vi "Wait.vi"(4 "error in (no error)":errorcluster, 6 "Delay (0ms)":i32 min=0 max=60000, 7 "VISA resource name":refnum<visa-resource-name>) -> (0 "error out":errorcluster, 3 "VISA resource name out":refnum<visa-resource-name>)   [LabVIEW 2015, in "Newport ESP301.lvlib"]
doc: "This command causes the controller to pause for a specified amount of time. This means that the controller will wait <B>Delay (0ms)</B> milliseconds before executing the next command.\nNote:\nEven though this command can be executed in immediate mode, its real value is as a flow control instruction inside programs.\nWait commands are primarily intended for use in internal program execution or in combination with the RQ command. If used in command mode, it is important to note that input command processing is suspended until the wait condition has been satisfied."
uses:
  Newport ESP301.lvlib
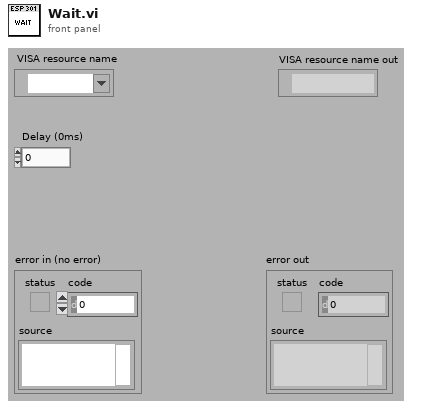
[diagram p1: front panel]
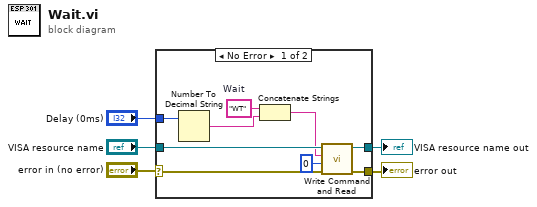
[diagram p0: block diagram]
diagram:
  n1 = case shown="No Error" "error in (no error)" {
    selector: "error in (no error)" -> [w11 w16]
    tunnel: [w13 w16] -> w5
    tunnel: "VISA resource name" -> [w14 w15]
    tunnel: [w12 w15] -> w4
    tunnel: "Delay (0ms)" -> [w8 _]
    frame No Error {
      w10 = "WT"  # Wait
      n2 = Number To Decimal String(number=w8) -> (decimal integer string=w6:string)  [unwired: 1 in]
      n3 = Concatenate Strings(w10, w6) -> (w9:string)
      n4 = call "Write Command and Read.vi"("error in (no error)"=w11, "Bytes to read (100)"=u32 0, "Command"=w9, "VISA resource name"=w14) -> ("error out"=w13:errorcluster, "VISA resource name out"=w12:refnum<visa-resource-name>)  [unwired: 3 in, 1 out]
    }
    frame Error {
    }
  }
  "error out" <- w5
  "VISA resource name out" <- w4
